vi "Scan DQMH Modules and create Maps.vi"(8 "error in":errorcluster, 10 "Include Dependencies":bool) -> (0 "error out":errorcluster, 1 "Tree Map out":T1, 2 "map ref out":map{string, refnum<vi>}(c390), 3 "DQMH Modules Info":T2)   [LabVIEW 2020, in "Panter Dashboard.lvlib"]
doc: "Gets the Singleton and Cloneable references and creates a list of each type of DQMH Modules"
uses:
  Panter Dashboard.lvlib
  DQMH Modules Info--cluster.ctl
  Module type--enum.ctl
  <vilib>/National Instruments/Tree Map/Tree Map Data.ctl
  <vilib>/National Instruments/Tree Map/Tree Map.lvlib
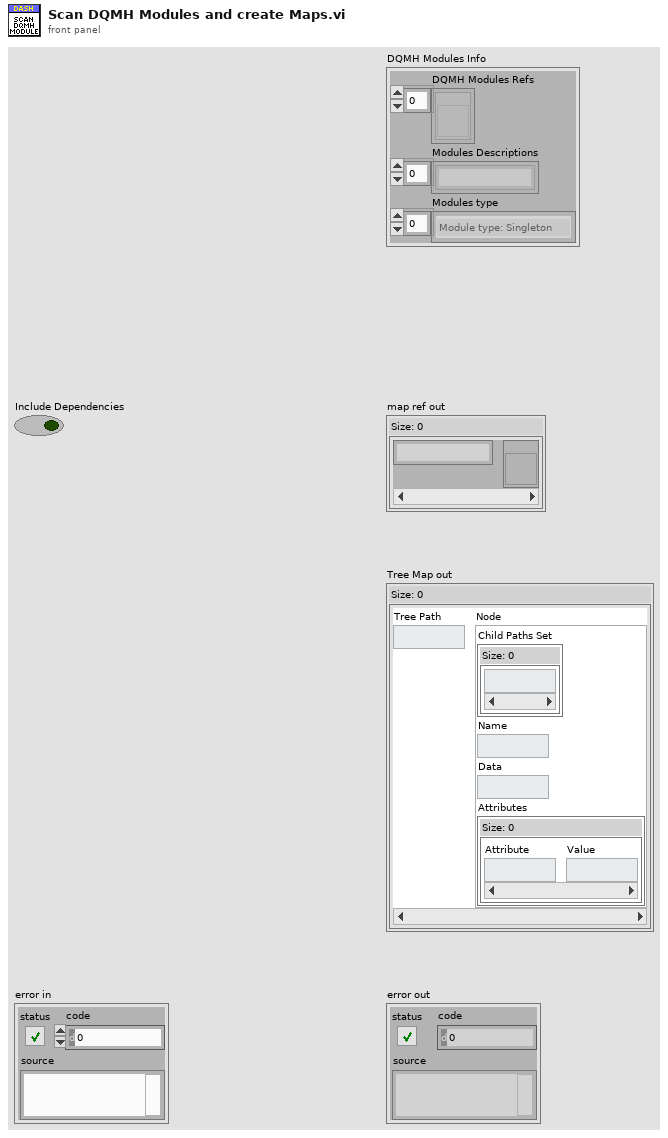
[diagram p1: front panel]
types:
  T1 = typedef "Tree Map.lvlib/Tree Map Data.ctl" = map{string, cluster{"Child Paths Set":set{string}, "Name":string, "Data":string, "Attributes":map{string, string}}}
  T2 = typedef "Panter Dashboard.lvlib/DQMH Modules Info--cluster.ctl" = cluster{"DQMH Modules Refs":refnum<vi>[], "Modules Descriptions":string[], "Modules type":T3[]}
  T3 = typedef "Panter Dashboard.lvlib/Module type--enum.ctl" = enum16{"Module type: Singleton", "Module type: Cloneable"}
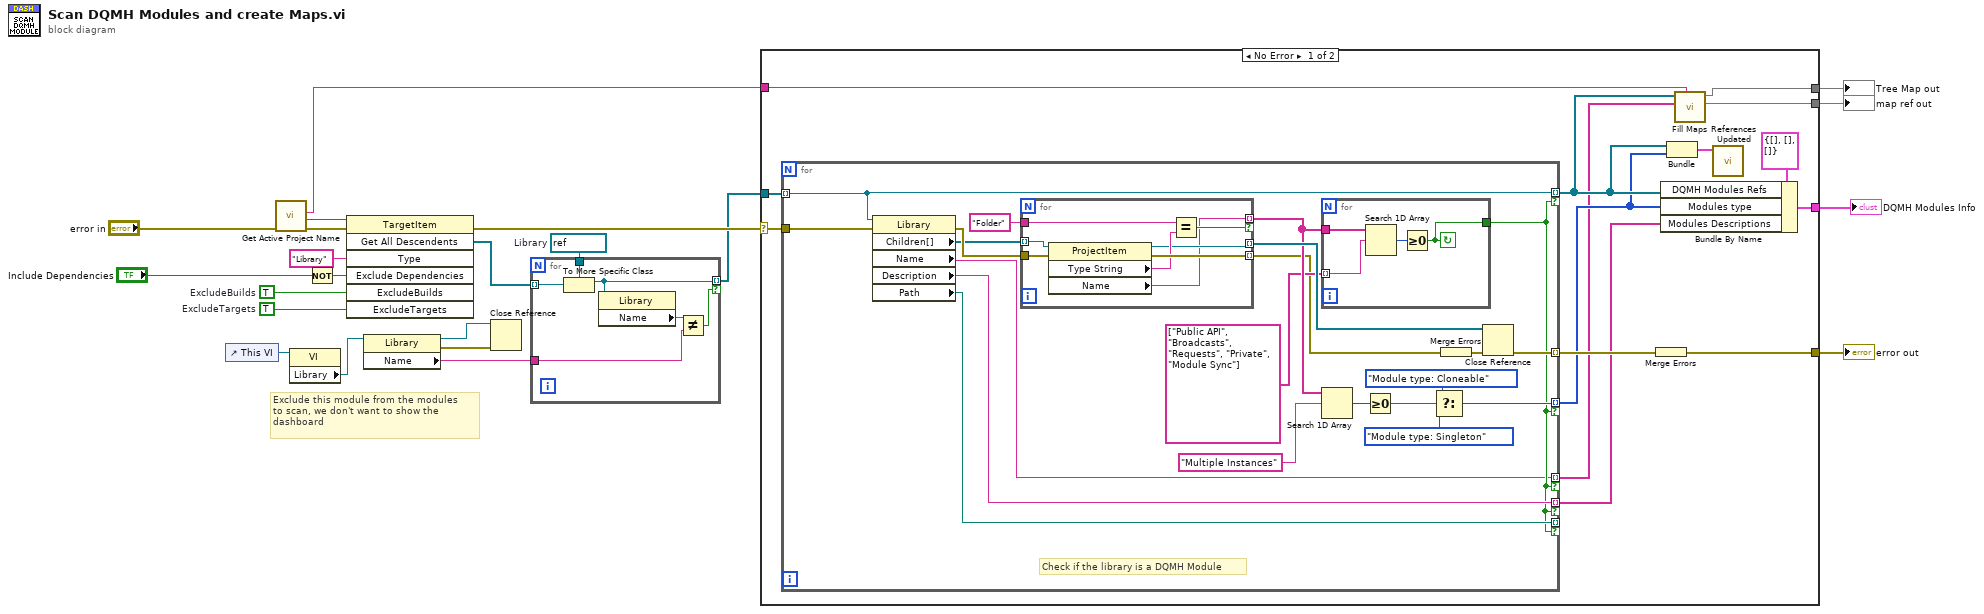
[diagram p0: block diagram]
diagram:
  w12 = refnum<vi> refnum  # Library
  w19 = TRUE  # ExcludeTargets
  w20 = TRUE  # ExcludeBuilds
  # "Exclude this module from the modules\nto scan, we don't want to show the\ndashboard"
  n1 = control-ref of="This VI"() -> (w7:refnum<vi>)
  n2 = call "Get Active Project Name.vi"("error in (no error)"="error in") -> ("error out"=w2:errorcluster, "Project Name"=w4:string, "Project Ref"=w5:refnum<vi>)  [unwired: 8 in]
  n3 = property class="VI"(reference=w7) -> ("Library"=w6:refnum<vi>)  [unwired: 1 in, 2 out]
  n4 = Not(x="Include Dependencies") -> (.not. x?=w15:bool)
  n5 = invoke class="TargetItem" method="Get All Descendents"(reference=w5, error in=w2, "Type"="Library", "Exclude Dependencies"=w15, "ExcludeBuilds"=w20, "ExcludeTargets"=w19) -> (error out=w22:errorcluster, "All Descendents"=w14:refnum<vi>[])  [unwired: 1 in, 5 out]
  n6 = property class="Library"(reference=w6) -> (reference out=w10:refnum<vi>, error out=w1:errorcluster, "Name"=w11:string)  [unwired: 1 in]
  n7 = Close Reference(reference=w10, error in (no error)=w1) -> ()  [unwired: 1 out]
  n8 = for {
    tunnel: w14 -> [w27] mode=indexing
    tunnel: [w23] -> w13 mode=indexing if=w28
    tunnel: w12 -> [w26]
    tunnel: w11 -> [w25]
    n9 = To More Specific Class(target class=w26, reference=w27) -> (specific class reference=w23:refnum<vi>)  [unwired: 1 in, 1 out]
    n10 = property class="Library"(reference=w23) -> ("Name"=w24:string)  [unwired: 1 in, 2 out]
    n11 = Not Equal?(x=w24, y=w25) -> (x != y?=w28:bool)
  }
  n12 = case shown="No Error" w22 {
    selector: w22 -> [w42 w76]
    tunnel: [w41 w76] -> w21
    tunnel: [w37 _] -> w16
    tunnel: w13 -> [w36 _]
    tunnel: [w35 _] -> w9
    tunnel: [w34 _] -> w8
    tunnel: w4 -> [w33 _]
    frame No Error {
      n13 = for {
        tunnel: [w61] -> w32 mode=indexing if=w57
        tunnel: w36 -> [w61] mode=indexing
        tunnel: [w63] -> w40 mode=indexing
        tunnel: w42 -> [w62]
        tunnel: [w60] -> w31 mode=indexing if=w57
        tunnel: [w56] -> w29 mode=indexing if=w57
        tunnel: [w59] -> w38 mode=indexing if=w57
        tunnel: [w58] -> _ mode=indexing if=w57
        # "Check if the library is a DQMH Module"
        n14 = property class="Library"(reference=w61, error in=w62) -> (error out=w55:errorcluster, "Children[]"=w52:refnum<vi>[], "Name"=w56:string, "Description"=w59:string, "Path"=w58:path)  [unwired: 1 out]
        n15 = for {
          tunnel: [w68] -> w48 mode=indexing if=w69
          tunnel: w55 -> [w75]
          tunnel: [w74] -> w46 mode=indexing
          tunnel: [w71] -> w51 mode=indexing
          tunnel: w52 -> [w73] mode=indexing
          tunnel: "Folder" ("Type") -> [w70]
          n16 = property class="ProjectItem"(reference=w73, error in=w75) -> (reference out=w71:refnum<vi>, error out=w74:errorcluster, "Type String"=w72:string, "Name"=w68:string)
          n17 = Equal?(x=w70, y=w72) -> (x = y?=w69:bool)
        }
        n18 = for {
          tunnel: string[] ["Public API", "Broadcasts", "Requests", "Private", "Module Sync"] -> [w67] mode=indexing
          tunnel: w48 -> [w66]
          tunnel: [w64] -> w57
          stop <- w64 continue-if-true
          n19 = Search 1D Array(1D array=w66, element=w67) -> (index of element=w65:i32)  [unwired: 1 in]
          n20 = Greater Or Equal To 0?(x=w65) -> (x >= 0?=w64:bool)
        }
        n21 = Search 1D Array(1D array=w48, element="Multiple Instances") -> (index of element=w50:i32)  [unwired: 1 in]
        n22 = Greater Or Equal To 0?(x=w50) -> (x >= 0?=w45:bool)
        n23 = Select(t=Module_type--enum."Module type: Cloneable", s=w45, f=Module_type--enum."Module type: Singleton" ("Module type")) -> (s? t:f=w60:T3)
        n24 = Merge Errors(w46) -> (w54:errorcluster)
        n25 = Close Reference(reference=w51, error in (no error)=w54) -> (error out=w63:errorcluster)
      }
      n26 = Merge Errors(w40) -> (w41:errorcluster)
      n27 = Bundle By Name(cluster=T2 {"DQMH Modules Refs"=[], "Modules Descriptions"=[], "Modules type"=[]} ("DQMH Modules Info"), "DQMH Modules Refs"=w32, "Modules type"=w31, "Modules Descriptions"=w38) -> (w37:T2)
      n28 = Bundle(w32, w31) -> (w30:cluster{refnum<vi>[], T3[]})  [unwired: 1 in]
      n29 = call "Fill Maps.vi"("Project Selected"=w33, "Module names"=w29, "DQMH Modules"=w32) -> ("map ref out"=w35:map{string, refnum<vi>}, "Tree Map out"=w34:T1)  [unwired: 7 in]
      n30 = call "References Updated.vi"("DQMH Refs"=w30) -> ()  [unwired: 10 in, 1 out]
    }
    frame Error {
    }
  }
  "error out" <- w21
  "DQMH Modules Info" <- w16
  "map ref out" <- w9
  "Tree Map out" <- w8
